vi "Main.vi"(8 "error in":errorcluster, 11 "Timer In":refnum<class "Timer.lvclass">) -> (0 "error out":errorcluster, 3 "Timer Out":refnum<class "Timer.lvclass">)   [LabVIEW 2021, in "Timer.lvclass"]
doc: "The <b>Queued Message Handler</b> of the Worker that owns this VI."
uses:
  Timer.lvclass
  Timer.lvclass/Timer.ctl
  <vilib>/ErrorRing/Error Ring.xnode
  <vilib>/addons/_Workers/Library/Case Label.ctl
  <vilib>/addons/_Workers/Library/Workers.lvlib
  rqp_Start.ctl
  <vilib>/Utility/error.llb/Error Cluster From Error Code.vi
  Timeout Settings.ctl
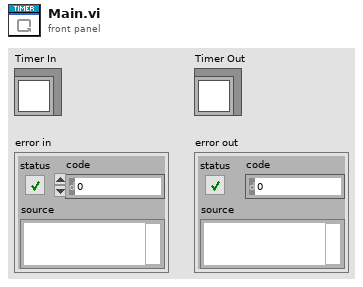
[diagram p1: front panel]
types:
  T1 = typedef "Timer.lvclass/Timeout Settings.ctl" = cluster{"Timeout (ms)":i32, "# Copies":i32}
  T2 = typedef "Timer.lvclass/rqp_Start.ctl" = cluster{"Timeout (ms)":i32, "# Copies":i32, "Response Case":T3}
  T3 = typedef "Workers.lvlib/Case Label.ctl" = string
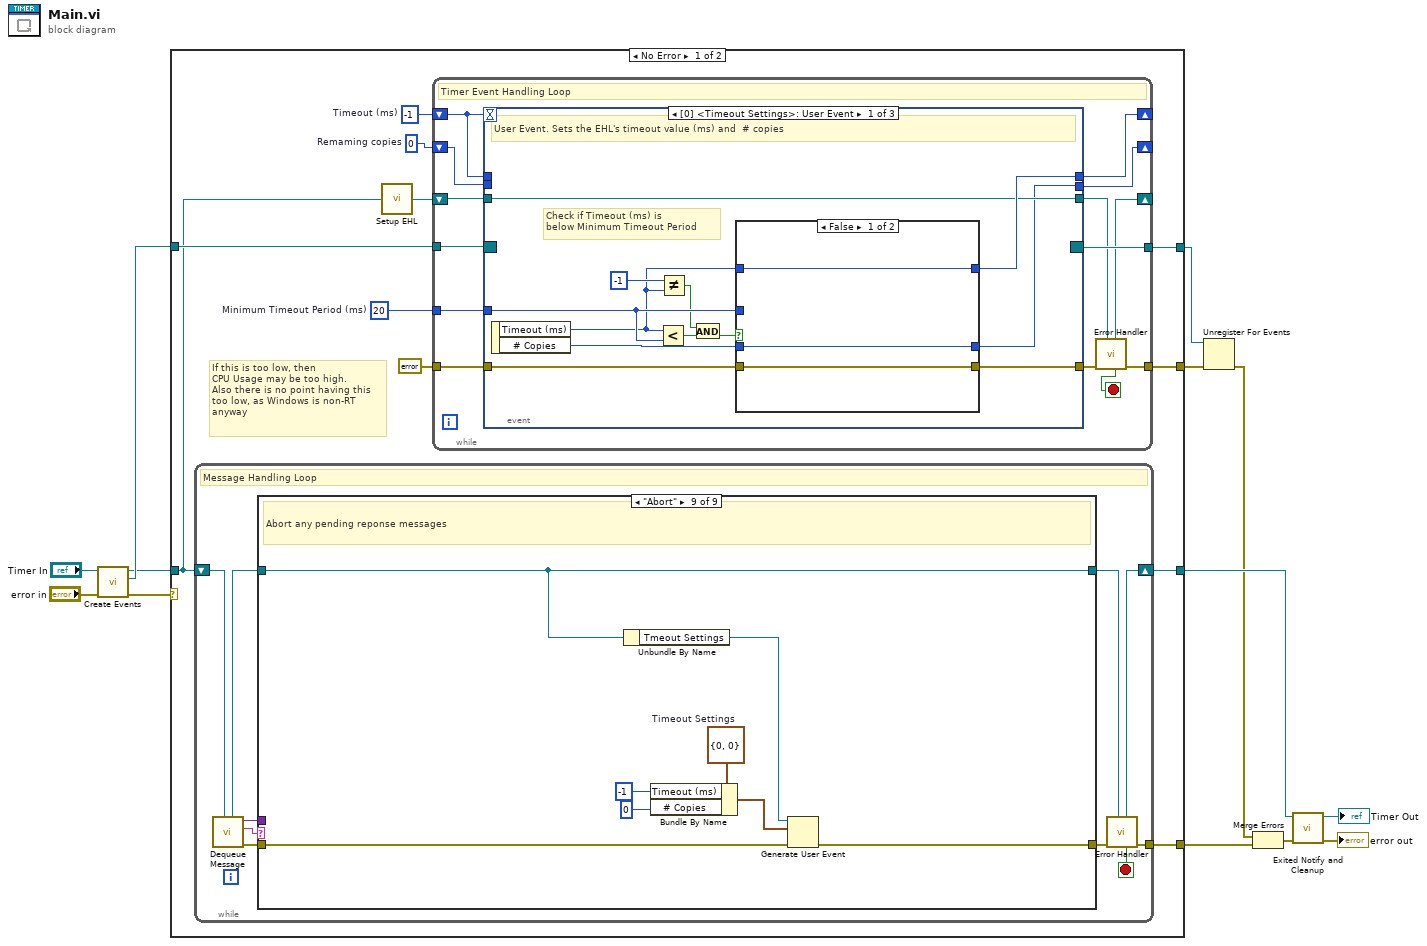
[diagram p0: block diagram]
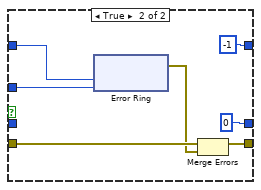
[diagram p2: hidden frame]
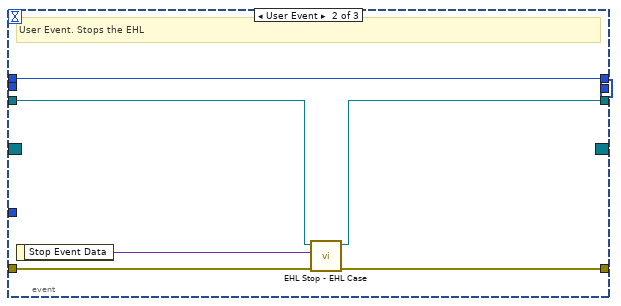
[diagram p3: hidden frame]
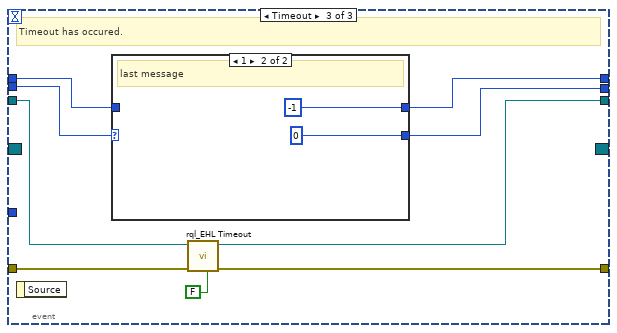
[diagram p4: hidden frame]
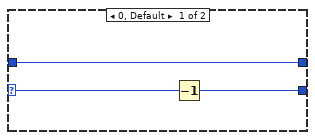
[diagram p5: hidden frame]
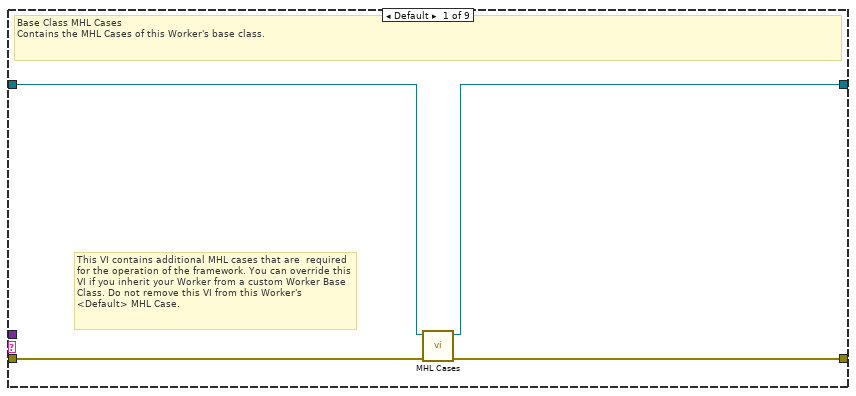
[diagram p6: hidden frame]
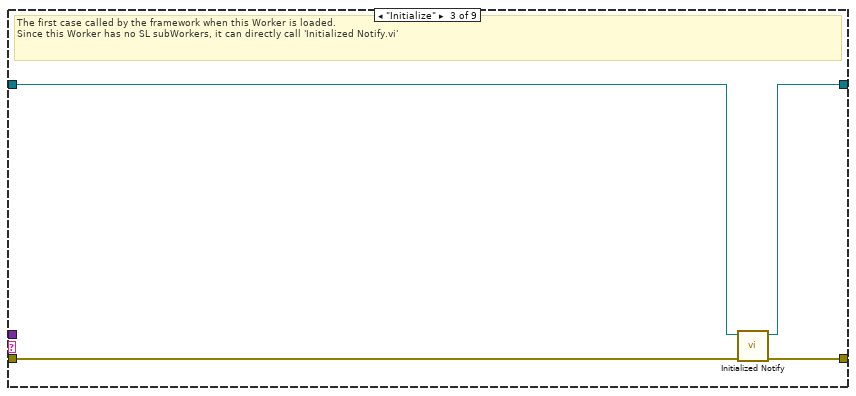
[diagram p8: hidden frame]
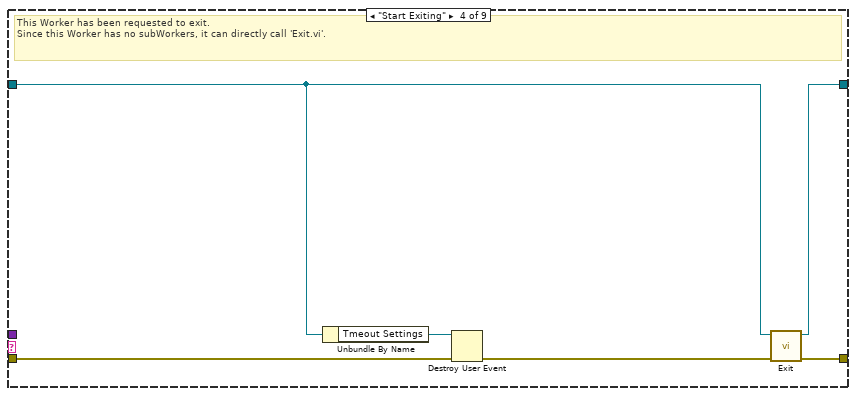
[diagram p9: hidden frame]
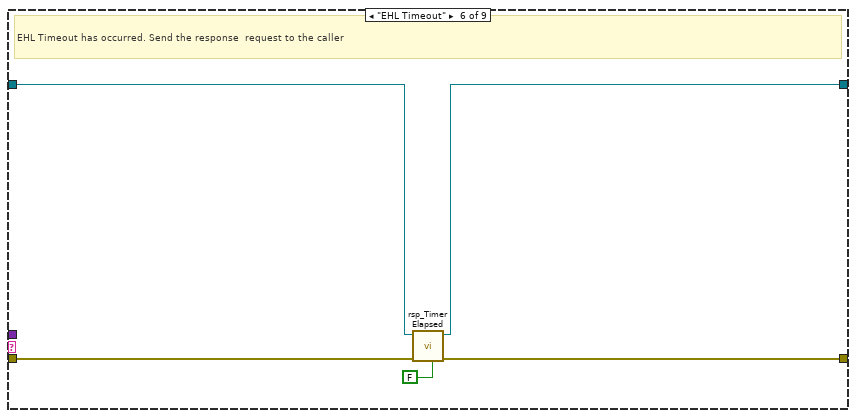
[diagram p11: hidden frame]
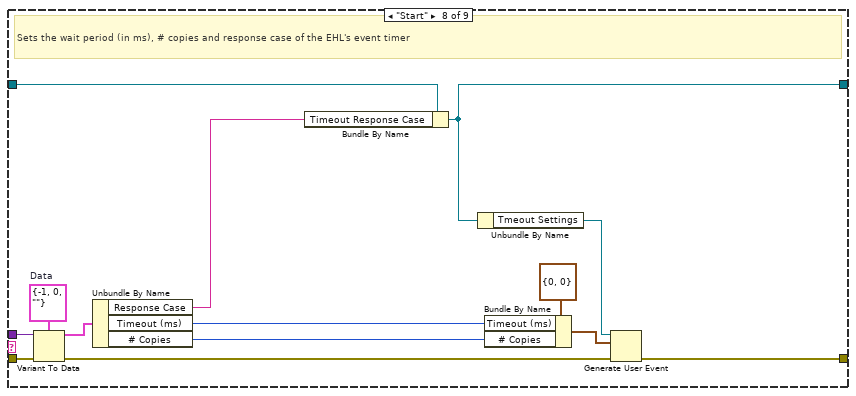
[diagram p13: hidden frame]
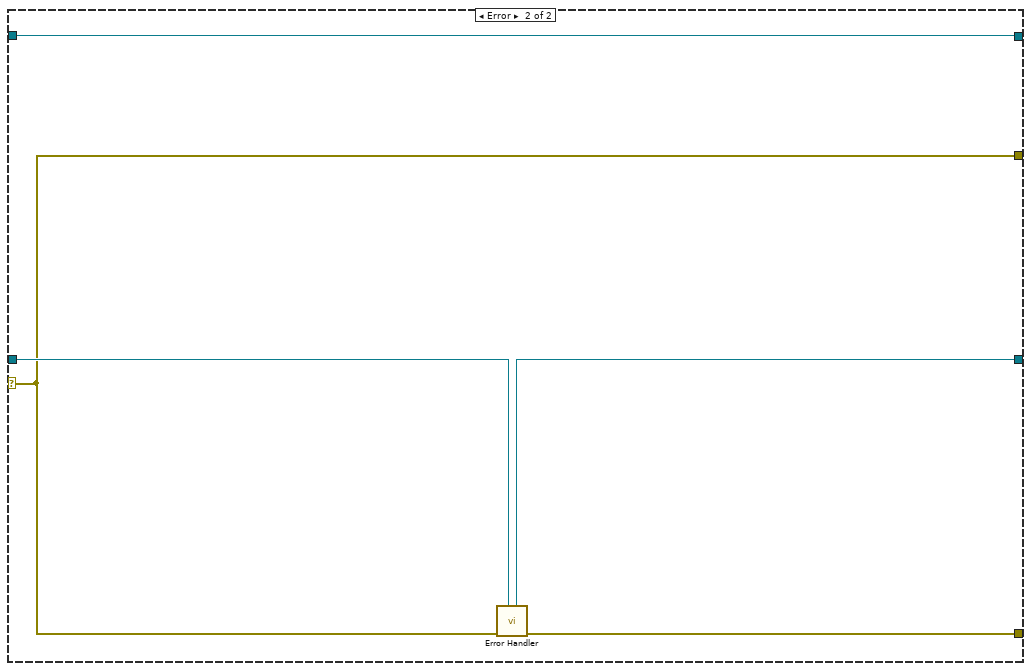
[diagram p14: hidden frame]
diagram:
  n1 = call "Create Events.vi"("error in"="error in", "Timer In"="Timer In") -> ("error out"=w8:errorcluster, "Event Registration Refnum"=w9:refnum<event-registration>, "Timer Out"=w4:refnum<class "Timer.lvclass">)  [unwired: 6 in]
  n2 = case shown="No Error" w8 {
    tunnel: w4 -> [w16 w150]
    tunnel: [w24 w151] -> w12
    tunnel: [w23 w149] -> w13
    selector: w8 -> [_ w148]
    tunnel: [w17 w148] -> w2
    tunnel: [w19 w147] -> w3
    tunnel: w9 -> [w18 w147]
    frame No Error {
      w14 = 0  # Remaming copies
      w22 = 20  # Minimum Timeout Period (ms)
      w21 = -1  # Timeout (ms)
      # "If this is too low, then \nCPU Usage may be too high.\nAlso there is no point having this\ntoo low, as Windows is non-RT\nanyway"
      n3 = while {
        shift-right: [w97] -> w23
        shift-left: w16 -> [w99]
        tunnel: [w98] -> w24
        stop <- w91 stop-if-true
        # "Message Handling Loop"
        n4 = call-dynamic "Dequeue Message.vi"("Worker"=w99) -> ("error out"=w96:errorcluster, "Case out"=w92:string, "Data out"=w90:variant, "Worker out"=w94:refnum<class "Timer.lvclass">)  [unwired: 6 in, 1 out]
        n5 = case "WORKERS MHL Case Structure (DO NOT CHANGE LABEL NAME)" shown="\"Abort\"" w92 {
          tunnel: w96 -> [w103 w104 w107 w111 w117 w122 w124 w138 w146]
          tunnel: [w102 w104 w109 w115 w117 w121 w124 w132 w142] -> w95
          tunnel: w94 -> [w101 w105 w106 w110 w116 w120 w123 w128 w141]
          tunnel: [w100 w105 w108 w114 w116 w119 w123 w127 w141] -> w93
          tunnel: w90 -> [_ _ _ _ _ _ _ w136 _]
          frame Default {
            # "This VI contains additional MHL cases that are  required for the operation of the framework. You can override this VI if you inherit your Worker from a custom Worker Base Class. Do not remove this VI from this Worker's <Default> MHL Case."
            # "Base Class MHL Cases\nContains the MHL Cases of this Worker's base class."
            n6 = call-dynamic "MHL Cases.vi"("error in"=w103, "Worker in"=w101) -> ("error out"=w102:errorcluster, "Worker out"=w100:refnum<class "Timer.lvclass">)  [unwired: 8 in]
          }
          frame "------------ FRAMEWORK CASES -----------" {
            # "Start of Workers Framework Cases"
          }
          frame "Initialize" {
            # "The first case called by the framework when this Worker is loaded.\nSince this Worker has no SL subWorkers, it can directly call 'Initialized Notify.vi'"
            n7 = call-dynamic "Initialized Notify.vi"("error in"=w107, "Worker"=w106) -> ("error out"=w109:errorcluster, "dup Worker out"=w108:refnum<class "Timer.lvclass">)  [unwired: 8 in]
          }
          frame "Start Exiting" {
            # "This Worker has been requested to exit.\nSince this Worker has no subWorkers, it can directly call 'Exit.vi'."
            n8 = Unbundle By Name(w110) -> ("Tmeout Settings"=w112:refnum<user-event>)
            n9 = Destroy User Event(user event=w112, error in=w111) -> (error out=w113:errorcluster)
            n10 = call-dynamic "Exit.vi"("error_in"=w113, "Worker"=w110) -> ("error out"=w115:errorcluster, "dup Worker out"=w114:refnum<class "Timer.lvclass">)  [unwired: 8 in]
          }
          frame "------------- LOCAL API CASES -------------" {
            # "Start of Workers Local API Cases"
          }
          frame "EHL Timeout" {
            # "EHL Timeout has occurred. Send the response  request to the caller"
            n11 = call "rsp_Timer Elapsed.vi"("Show in Debugger?"=FALSE, "error in"=w122, "Timer In"=w120) -> ("error out"=w121:errorcluster, "Timer Out"=w119:refnum<class "Timer.lvclass">)  [unwired: 7 in]
          }
          frame "------------- PUBLIC API CASES -------------" {
            # "Start of Workers Public API Cases"
          }
          frame "Start" {
            w137 = T2 {"Timeout (ms)"=-1, "# Copies"=0, "Response Case"=""}  # Data
            # "Sets the wait period (in ms), # copies and response case of the EHL's event timer"
            n12 = Variant To Data(error in=w138, type=w137, Variant=w136) -> (data=w135:T2, error out=w133:errorcluster)
            n13 = Unbundle By Name(w135) -> ("Response Case"=w126:T3, "Timeout (ms)"=w130:i32, "# Copies"=w129:i32)
            n14 = Bundle By Name(cluster=w128, "Timeout Response Case"=w126) -> (w127:refnum<class "Timer.lvclass">)
            n15 = Unbundle By Name(w127) -> ("Tmeout Settings"=w134:refnum<user-event>)
            n16 = Bundle By Name(cluster=T1 {"Timeout (ms)"=0, "# Copies"=0} ("Setting Timeout(s)"), "Timeout (ms)"=w130, "# Copies"=w129) -> (w131:T1)
            n17 = Generate User Event(user event=w134, event data cluster=w131, error in=w133) -> (error out=w132:errorcluster)  [unwired: 1 in, 1 out]
          }
          frame "Abort" {
            w144 = T1 {"Timeout (ms)"=0, "# Copies"=0}  # Timeout Settings
            # "Abort any pending reponse messages"
            n18 = Unbundle By Name(w141) -> ("Tmeout Settings"=w145:refnum<user-event>)
            n19 = Bundle By Name(cluster=w144, "Timeout (ms)"=-1 ("Set Timeout (ms)"), "# Copies"=0) -> (w143:T1)
            n20 = Generate User Event(user event=w145, event data cluster=w143, error in=w146) -> (error out=w142:errorcluster)  [unwired: 1 in, 1 out]
          }
        }
        n21 = call-dynamic "Error Handler.vi"("Worker"=w93, "error_in"=w95) -> ("error out"=w98:errorcluster, "Stop Loop"=w91:bool, "Worker out"=w97:refnum<class "Timer.lvclass">)  [unwired: 7 in]
      }
      n22 = call-dynamic "Setup EHL.vi"("Worker"=w16) -> ("Worker out"=w15:refnum<class "Timer.lvclass">)  [unwired: 14 in]
      n23 = while "Event Handling Loop" {
        shift-right: [w27] -> _
        shift-left: w21 -> [w37]
        tunnel: errorcluster {"status"=FALSE, "code"=0, "source"=""} ("error IO") -> [w38]
        tunnel: [w32] -> w17
        tunnel: w18 -> [w36]
        tunnel: [w35] -> w19
        tunnel: w22 -> [w34]
        shift-right: [w29] -> _
        shift-left: w15 -> [w31]
        shift-right: [w26] -> _
        shift-left: w14 -> [w25]
        stop <- w28 stop-if-true
        # "Timer Event Handling Loop"
        n24 = event shown="[0] <Timeout Settings>: User Event" {
          selector: w36 -> [_ _ _]
          dyn-events: [_ _ _] -> w35
          timeout: w37 -> [_ _ _]
          tunnel: w38 -> [w48 w75 w84]
          tunnel: [w49 w73 w83] -> w33
          tunnel: w37 -> [_ w74 w76]
          tunnel: [w46 w74 w77] -> w27
          tunnel: w34 -> [w47 _ _]
          tunnel: w31 -> [w41 w72 w82]
          tunnel: [w41 w71 w81] -> w30
          tunnel: [w40 0 ("Remaming copies") w78] -> w26
          tunnel: w25 -> [_ _ w79]
          event User Event {
            # "Check if Timeout (ms) is\nbelow Minimum Timeout Period"
            # "User Event. Sets the EHL's timeout value (ms) and  # copies"
            n25 = event-data() -> ("Timeout (ms)"=w43:i32, "# Copies"=w39:i32)  [unwired: 1 in]
            n26 = Less?(x=w43, y=w47) -> (x < y?=w50:bool)
            n27 = Not Equal?(x=-1 ("Set Timeout (ms)"), y=w43) -> (x != y?=w42:bool)
            n28 = And(x=w42, y=w50) -> (x .and. y?=w45:bool)
            n29 = case shown="False" w45 {
              tunnel: [w53 w58] -> w49
              tunnel: w48 -> [w53 w59]
              tunnel: w43 -> [w52 w56]
              tunnel: w47 -> [_ w55]
              tunnel: [w52 -1 ("Set Timeout (ms)")] -> w46
              tunnel: [w51 0 ("Set Timeout (ms)")] -> w40
              tunnel: w39 -> [w51 _]
              frame False {
              }
              frame True {
                n30 = xnode "Error Ring"("parameter 0"=w56, "parameter 1"=w55) -> ("error out"=w57:errorcluster)
                n31 = Merge Errors(w59, w57) -> (w58:errorcluster)
              }
            }
          }
          event User Event {
            # "User Event. Stops the EHL"
            n32 = event-data() -> ("Stop Event Data"=w70:variant)  [unwired: 1 in]
            n33 = call-dynamic "EHL Stop - EHL Case.vi"("error in"=w75, "Stop Event Data"=w70, "Worker"=w72) -> ("error out"=w73:errorcluster, "Worker out"=w71:refnum<class "Timer.lvclass">)  [unwired: 7 in]
          }
          event Timeout {
            # "Timeout has occured."
            n34 = event-data() -> ()  [unwired: 1 in, 1 out]
            n35 = case shown="1" w79 {
              selector: w79 -> [w87 _]
              tunnel: [w86 0] -> w78
              tunnel: [w85 -1 ("Timeout (ms)")] -> w77
              tunnel: w76 -> [w85 _]
              frame 0, Default {
                n36 = Decrement(x=w87) -> (x-1=w86:i32)
              }
              frame 1 {
                # "last message"
              }
            }
            n37 = call "rql_EHL Timeout.vi"("Show in Debugger?"=FALSE, "error in"=w84, "Timer In"=w82) -> ("error out"=w83:errorcluster, "Timer Out"=w81:refnum<class "Timer.lvclass">)  [unwired: 7 in]
          }
        }
        n38 = call-dynamic "Error Handler.vi"("Worker"=w30, "error_in"=w33) -> ("error out"=w32:errorcluster, "Stop Loop"=w28:bool, "Worker out"=w29:refnum<class "Timer.lvclass">)  [unwired: 7 in]
      }
    }
    frame Error {
      n39 = call-dynamic "Error Handler.vi"("Worker"=w150, "error_in"=w148) -> ("error out"=w151:errorcluster, "Worker out"=w149:refnum<class "Timer.lvclass">)  [unwired: 7 in, 1 out]
    }
  }
  n40 = Unregister For Events(event registration refnum=w3, error in=w2) -> (error out=w1:errorcluster)
  n41 = Merge Errors(w1, w12) -> (w11:errorcluster)
  n42 = call-dynamic "Exited Notify and Cleanup.vi"("error_in"=w11, "Worker"=w13) -> ("error out"=→"error out":errorcluster, "dup Worker out"=→"Timer Out":refnum<class "Timer.lvclass">)  [unwired: 8 in]
